vi "Log Prompt UI.vi"(9 "Target Prompt":string, 10 "Group Prompt":string) -> (1 "Cancelled":bool, 2 "Series":string)   [LabVIEW 2020, in "VolatusGUIElements.lvlib" / "GroupLoggingControl.lvclass"]
uses:
  GroupLoggingControl.lvclass
  GroupLoggingControl.lvclass/GroupLoggingControl.ctl
  <vilib>/Utility/miscctls.llb/LVSelectionTypeDef.ctl
  <vilib>/regexp/Match Regular Expression.xnode
panel:
  in  "Series Input":string
  in  "Cancel":bool
  in  "Accept":bool
  # "Enter log series name to begin logging:"
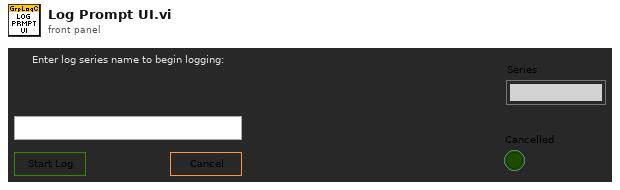
[diagram p1: front panel]
types:
  T1 = enum8{"Enabled", "Disabled", "Disabled and Grayed Out"}
  T2 = typedef "LVSelectionTypeDef.ctl" = cluster{"Selection Start":u32, "Selection End":u32}
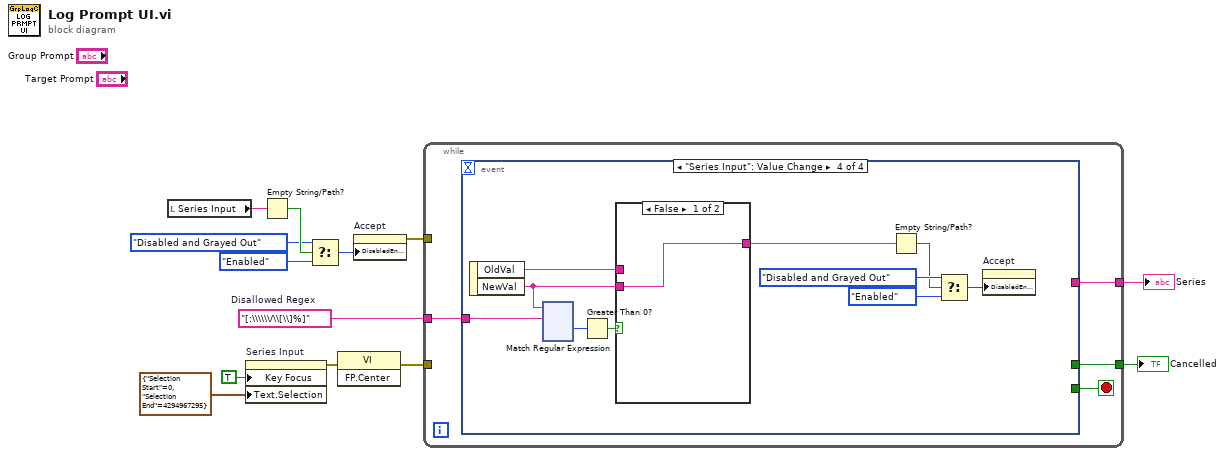
[diagram p0: block diagram]
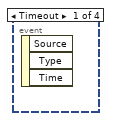
[diagram p2: hidden frame]
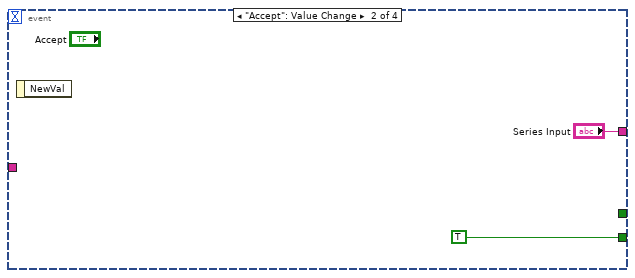
[diagram p3: hidden frame]
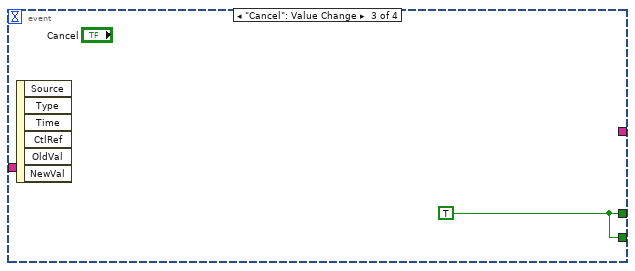
[diagram p4: hidden frame]
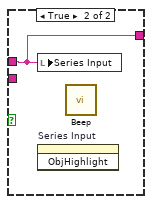
[diagram p5: hidden frame]
diagram:
  w7 = "[:\\\\\\/\\[\\]%]"  # Disallowed Regex
  n1 = local read "Series Input"() -> (w1:string)
  n2 = property on="Series Input" class="Str"("Key Focus"=TRUE, "Text.Selection"=T2 {"Selection Start"=0, "Selection End"=4294967295}) -> (error out=w11:errorcluster)  [unwired: 2 in, 1 out]
  n3 = Empty String/Path?(string/path=w1) -> (empty?=w5:bool)
  n4 = Select(t=T1."Disabled and Grayed Out" ("Disabled"), s=w5, f=T1."Enabled" ("Disabled")) -> (s? t:f=w6:T1)
  n5 = invoke class="VI" method="FP.Center"(error in=w11) -> (error out=w10:errorcluster)  [unwired: 2 in, 2 out]
  n6 = property on="Accept" class="Bool"("DisabledEnum"=w6) -> (error out=w2:errorcluster)  [unwired: 2 in, 1 out]
  n7 = while {
    tunnel: w10 -> [_]
    tunnel: [w16] -> w9
    tunnel: [w15] -> w8
    tunnel: w7 -> [w14]
    tunnel: w2 -> [_]
    stop <- w17 stop-if-true
    n8 = event shown="[3] \"Series Input\": Value Change" {
      selector: _ -> [_ _ _ _]
      dyn-events: _ -> [_ _ _ _]
      timeout: _ -> [_ _ _ _]
      tunnel: [_ TRUE w20 _] -> w17
      tunnel: [_ _ w20 _] -> w16
      tunnel: [_ "Series Input" _ _] -> w15
      tunnel: w14 -> [_ _ _ w30]
      event Timeout {
        n9 = event-data() -> ()  [unwired: 1 in, 3 out]
      }
      event "Accept": Value Change {
        n10 = event-data() -> ()  [unwired: 1 in, 1 out]
      }
      event "Cancel": Value Change {
        w20 = TRUE
        n11 = event-data() -> ()  [unwired: 1 in, 6 out]
      }
      event "Series Input": Value Change {
        n12 = event-data() -> ("OldVal"=w27:string, "NewVal"=w26:string)  [unwired: 1 in]
        n13 = xnode "Match Regular Expression"("input string"=w26, "regular expression"=w30) -> ("offset past match"=w29:i32)  [unwired: 4 in, 4 out]
        n14 = Greater Than 0?(x=w29) -> (x > 0?=w28:bool)
        n15 = case shown="False" w28 {
          tunnel: w27 -> [_ w32]
          tunnel: w26 -> [w31 _]
          tunnel: [w31 w32] -> w25
          frame False {
          }
          frame True {
            n16 = local write "Series Input"(w32) -> ()
            n17 = invoke on="Series Input" class="Str" method="ObjHighlight"() -> ()  [unwired: 3 in, 3 out]
            n18 = call <vilib>:"Beep.vi"() -> ()  [unwired: 12 in]
          }
        }
        n19 = Empty String/Path?(string/path=w25) -> (empty?=w22:bool)
        n20 = Select(t=T1."Disabled and Grayed Out" ("Disabled"), s=w22, f=T1."Enabled" ("Disabled")) -> (s? t:f=w21:T1)
        n21 = property on="Accept" class="Bool"("DisabledEnum"=w21) -> ()  [unwired: 2 in, 2 out]
      }
    }
  }
  "Series" <- w8
  "Cancelled" <- w9
